vi "setData.vi"(10 "T7InclinometerData":T1, 11 "T7Inclinometer in":refnum<class "T7Inclinometer.lvclass">) -> (3 "T7Inclinometer out":refnum<class "T7Inclinometer.lvclass">)   [LabVIEW 2016, in "RTT7Inclinometer.lvlib" / "T7Inclinometer.lvclass"]
uses:
  T7Inclinometer.lvclass
  DataTypes/T7InclinometerData.ctl
  DataTypes/T7InclinometerConstants.ctl
  DataTypes/T7InclinometerTelemetry.ctl
  DataTypes/T7InclinometerResponses.ctl
  DataTypes/T7InclinometerErrors.ctl
  DataTypes/T7InclinometerTimestamps.ctl
  T7Inclinometer.lvclass/T7Inclinometer.ctl
  RTT7Inclinometer.lvlib
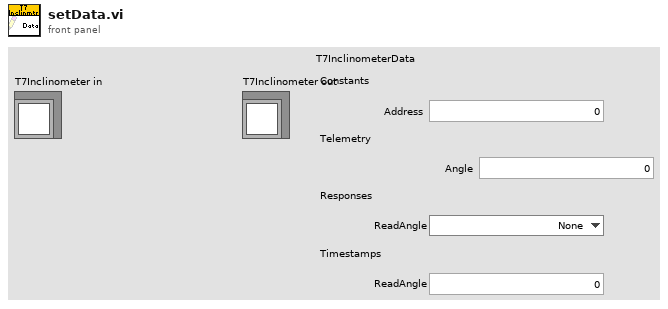
[diagram p1: front panel]
types:
  T1 = typedef "RTT7Inclinometer.lvlib/T7InclinometerData.ctl" = cluster{"Constants":T2, "Telemetry":T3, "Responses":T4, "Timestamps":T6}
  T2 = typedef "RTT7Inclinometer.lvlib/T7InclinometerConstants.ctl" = cluster{"Address":u8}
  T3 = typedef "RTT7Inclinometer.lvlib/T7InclinometerTelemetry.ctl" = cluster{"Angle":dbl}
  T4 = typedef "RTT7Inclinometer.lvlib/T7InclinometerResponses.ctl" = cluster{"ReadAngle":T5}
  T5 = typedef "RTT7Inclinometer.lvlib/T7InclinometerErrors.ctl" = enum16{"None", "InvalidFunctionCodeError", "InvalidRegisterAddressError", "InvalidCRCError", "UnknownAddressError", "UnknownFunctionError", "InvalidResponseLengthError", "UnknownError"}
  T6 = typedef "RTT7Inclinometer.lvlib/T7InclinometerTimestamps.ctl" = cluster{"ReadAngle":dbl}
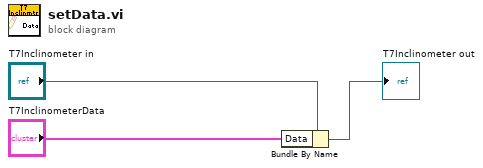
[diagram p0: block diagram]
diagram:
  n1 = Bundle By Name(cluster="T7Inclinometer in", "Data"="T7InclinometerData") -> (→"T7Inclinometer out":refnum<class "T7Inclinometer.lvclass">)
